vi "Set_RAW.vi"(0 "reference in":refnum<class "AI.lvclass">, 5 "RAW":dbl, 11 "error in (no error)":errorcluster) -> (4 "reference out":refnum<class "AI.lvclass">, 15 "error out":errorcluster)   [LabVIEW 2019, in "AI.lvclass"]
uses:
  AI.lvclass
  AI.lvclass/AI.ctl
  AnalogComparator_class/AnalogComparator.lvclass/AnalogComparator.ctl
  AnalogComparator_class/SetValue.vi
  AnalogComparator_class/HandleDb.vi
  Scale_class/Scale.lvclass
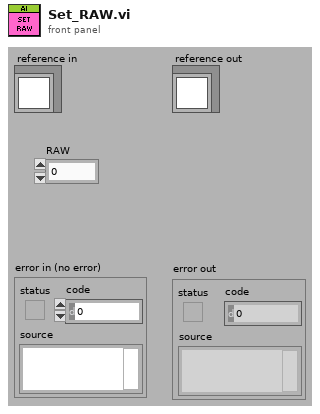
[diagram p1: front panel]
types:
  T1 = typedef "Data Avr.ctl" = cluster{"data":dbl[]}
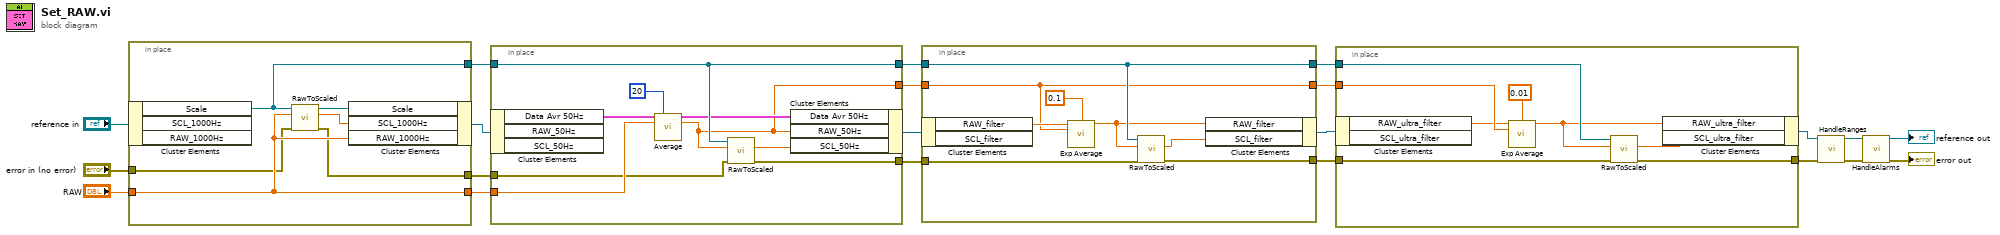
[diagram p0: block diagram]
diagram:
  n1 = in-place {
    in-place-border: "RAW" -> [w26]
    in-place-border: [w26] -> w11
    in-place-border: "error in (no error)" -> [w25]
    in-place-border: [w24] -> w9
    in-place-border: [w22] -> w5
    n2 = in-place-cluster #1("reference in") -> ("Scale"=w22:refnum<class "Scale.lvclass">)  [unwired: 2 out]
    n3 = call-dynamic "RawToScaled.vi"("error in (no error)"=w25, "RAW"=w26, "Scale in"=w22) -> ("error out"=w24:errorcluster, "Scaled"=w27:dbl, "Scale out"=w23:refnum<class "Scale.lvclass">)  [unwired: 6 in]
    n4 = in-place-cluster #1("Scale"=w23, "SCL_1000Hz"=w27, "RAW_1000Hz"=w26) -> (w12:refnum<class "AI.lvclass">)
  }
  n5 = in-place {
    in-place-border: w11 -> [w36]
    in-place-border: w9 -> [w34]
    in-place-border: [w33] -> w8
    in-place-border: [w32] -> w4
    in-place-border: w5 -> [w32]
    in-place-border: [w28] -> w2
    n6 = in-place-cluster #2(w12) -> ("Data Avr 50Hz"=w31:T1)  [unwired: 2 out]
    n7 = call "Average.vi"("Data Avr in"=w31, "Size"=20, "VALUE"=w36) -> ("Data Avr out"=w30:T1, "AVR"=w28:dbl)  [unwired: 11 in]
    n8 = call-dynamic "RawToScaled.vi"("error in (no error)"=w34, "RAW"=w28, "Scale in"=w32) -> ("error out"=w33:errorcluster, "Scaled"=w35:dbl)  [unwired: 6 in, 1 out]
    n9 = in-place-cluster #2("Data Avr 50Hz"=w30, "RAW_50Hz"=w28, "SCL_50Hz"=w35) -> (w17:refnum<class "AI.lvclass">)
  }
  n10 = in-place {
    in-place-border: w8 -> [w43]
    in-place-border: [w42] -> w7
    in-place-border: w4 -> [w41]
    in-place-border: [w41] -> w3
    in-place-border: w2 -> [w37]
    in-place-border: [w37] -> w1
    n11 = in-place-cluster #3(w17) -> ("RAW_filter"=w40:dbl)  [unwired: 1 out]
    n12 = call "Exp Average.vi"("s[i -1]"=w40, "alfa"=0.1, "x"=w37) -> ("s[i]"=w38:dbl)  [unwired: 12 in]
    n13 = call-dynamic "RawToScaled.vi"("error in (no error)"=w43, "RAW"=w38, "Scale in"=w41) -> ("error out"=w42:errorcluster, "Scaled"=w44:dbl)  [unwired: 6 in, 1 out]
    n14 = in-place-cluster #3("RAW_filter"=w38, "SCL_filter"=w44) -> (w16:refnum<class "AI.lvclass">)
  }
  n15 = in-place {
    in-place-border: w7 -> [w51]
    in-place-border: [w50] -> w6
    in-place-border: w3 -> [w49]
    in-place-border: w1 -> [w47]
    n16 = in-place-cluster #4(w16) -> ("RAW_ultra_filter"=w46:dbl)  [unwired: 1 out]
    n17 = call "Exp Average.vi"("s[i -1]"=w46, "alfa"=0.01, "x"=w47) -> ("s[i]"=w45:dbl)  [unwired: 12 in]
    n18 = call-dynamic "RawToScaled.vi"("error in (no error)"=w51, "RAW"=w45, "Scale in"=w49) -> ("error out"=w50:errorcluster, "Scaled"=w52:dbl)  [unwired: 6 in, 1 out]
    n19 = in-place-cluster #4("RAW_ultra_filter"=w45, "SCL_ultra_filter"=w52) -> (w15:refnum<class "AI.lvclass">)
  }
  n20 = call "HandleRanges.vi"("reference in"=w15, "error in (no error)"=w6) -> ("reference out"=w19:refnum<class "AI.lvclass">, "error out"=w18:errorcluster)  [unwired: 12 in]
  n21 = call "HandleAlarms.vi"("reference in"=w19, "error in (no error)"=w18) -> ("reference out"=→"reference out":refnum<class "AI.lvclass">, "error out"=→"error out":errorcluster)  [unwired: 12 in]
